vi "StringToMatrix.vi"(9 "String In":string, 10 "Number of Rows":i32, 11 "Number of Columns":i32) -> (3 "Matrix Out":T1)   [LabVIEW 2014]
uses:
  <vilib>/Analysis/Matrix/Datatypes/RealMatrix.ctl
  <vilib>/Analysis/Matrix/NI_Matrix.lvlib
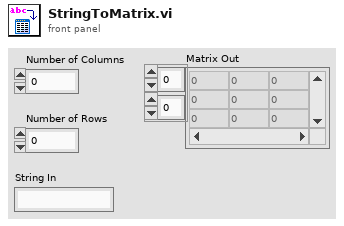
[diagram p1: front panel]
types:
  T1 = typedef "NI_Matrix.lvlib/RealMatrix.ctl" = dbl[][]
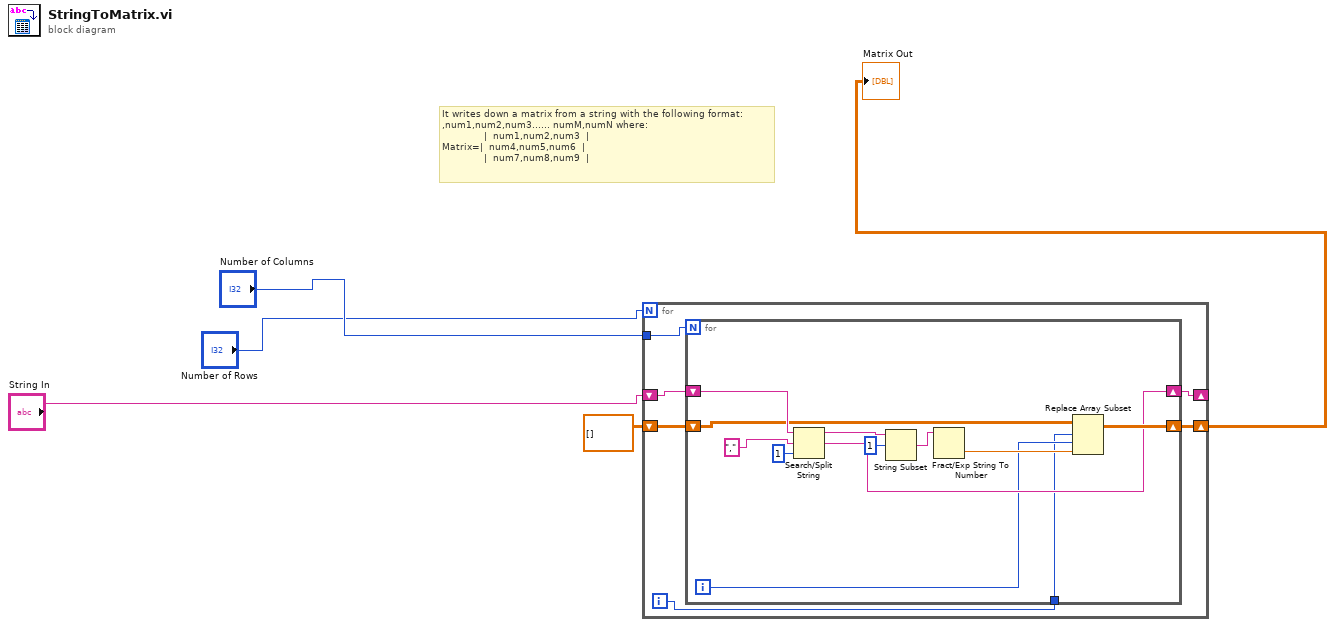
[diagram p0: block diagram]
diagram:
  # "It writes down a matrix from a string with the following format:\n,num1,num2,num3...... numM,numN where:\n              |  num1,num2,num3  |\nMatrix=|  num4,num5,num6  |\n              |  num7,num8,num9  |"
  n1 = for {
    N: "Number of Rows" -> [_]
    shift-right: [w9] -> w5
    shift-left: T1 [] ("Real Matrix") -> [w8]
    shift-right: [w7] -> _
    shift-left: "String In" -> [w11]
    tunnel: "Number of Columns" -> [w6]
    i -> [w10]
    n2 = for {
      N: w6 -> [_]
      tunnel: w10 -> [w12]
      shift-right: [w19] -> w9
      shift-left: w8 -> [w18]
      shift-right: [w17] -> w7
      shift-left: w11 -> [w23]
      i -> [w13]
      n3 = Search/Split String(string=w23, search string/char (-)=",", offset (0)=1) -> (substring before match=w16:string, match + rest of string=w17:string)  [unwired: 1 out]
      n4 = String Subset(string=w16, offset (0)=1) -> (substring=w15:string)  [unwired: 1 in]
      n5 = Fract/Exp String To Number(string=w15) -> (number=w20:dbl)  [unwired: 3 in, 1 out]
      n6 = Replace Array Subset(array=w18, new element=w20, index (row)=w12, index (col)=w13) -> (w19:T1)
    }
  }
  "Matrix Out" <- w5
